vi "Query Status Register.vi"(8 "error in":errorcluster, 11 "57XX in":refnum<class "57XX.lvclass">) -> (0 "error out":errorcluster, 3 "57XX out":refnum<class "57XX.lvclass">)   [LabVIEW 2019, in "57XX.lvlib" / "57XX.lvclass"]
doc: "Child classes must override this VI:\n\nThis VI is the device specific query of the supply's status registers. \nThe return values are: \n\nThe implementation must read status registers and push the status register values to private data for:\nOCP Flag, OVP Flag, Interlock Flag, Output Flag into the private data arrays of the power supply class."
uses:
  Library/57XX.lvclass
  C:/Users/Public/Documents/Development/builds/Instruments/PowerSupply.lvlibp/Library/PowerSupply.lvclass
  builds/Instruments/PowerSupply.lvlibp/Custom Controls/Status_Flags.ctl
  builds/Instruments/PowerSupply.lvlibp/Accessors/Write Status Flags.vi
  builds/Instruments/PowerSupply.lvlibp/Library/PowerSupply.lvclass
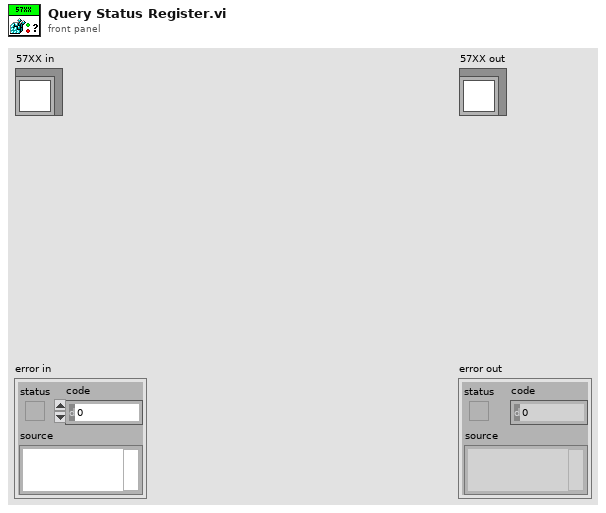
[diagram p1: front panel]
types:
  T1 = typedef "PowerSupply.lvlibp/PowerSupply.lvclass/Status_Flags.ctl" = cluster{"Interlock":bool, "OVP":bool, "OCP":bool, "Output":bool}
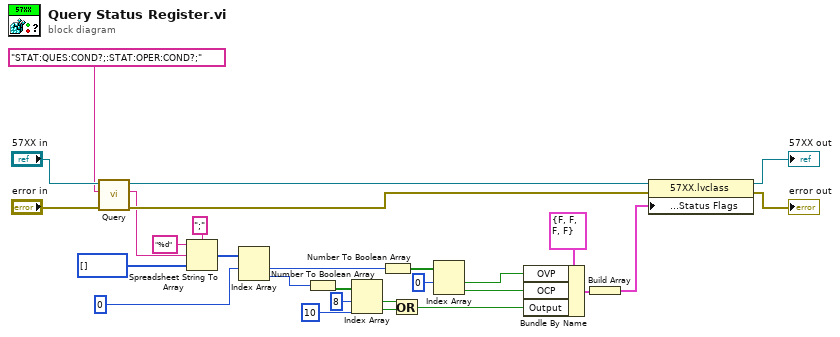
[diagram p0: block diagram]
diagram:
  n1 = call "Query.vi"("error in"="error in", "Write in"="STAT:QUES:COND?;:STAT:OPER:COND?;", "57XX in"="57XX in") -> ("error out"=w21:errorcluster, "Read out"=w4:string, "57XX out"=w24:refnum<class "57XX.lvclass">)  [unwired: 6 in]
  n2 = Spreadsheet String To Array(delimiter (Tab)=";", format string="%d", spreadsheet string=w4, array type (2D Dbl)=i32[] []) -> (array=w6:i32[])
  n3 = Index Array(array=w6, index #1=0 ("index")) -> (element #1=w3:i32, element #2=w2:i32)  [unwired: 1 in]
  n4 = Number To Boolean Array(number=w2) -> (Boolean array=w20:bool[])
  n5 = Index Array(array=w20, index #1=8 ("index"), index #2=10 ("index")) -> (element #1=w19:bool, element #2=w18:bool)
  n6 = Number To Boolean Array(number=w3) -> (Boolean array=w13:bool[])
  n7 = Or(x=w19, y=w18) -> (x .or. y?=w17:bool)
  n8 = Index Array(array=w13, index #1=0 ("index")) -> (element #1=w11:bool, element #2=w10:bool)  [unwired: 1 in]
  n9 = Bundle By Name(cluster=T1 {"Interlock"=FALSE, "OVP"=FALSE, "OCP"=FALSE, "Output"=FALSE} ("Status"), "OVP"=w11, "OCP"=w10, "Output"=w17) -> (w25:T1)
  n10 = Build Array(w25) -> (w14:T1[])
  n11 = property class="57XX.lvclass"(reference=w24, error in=w21, "Accessors:GUI:Status:Status Flags"=w14) -> (reference out=→"57XX out":refnum<class "57XX.lvclass">, error out=→"error out":errorcluster)
